vi "streams test.vi"() -> ()   [LabVIEW 2013, in "tag bus tests.lvlib"]
uses:
  tag bus tests.lvlib
  data stream/publisher/publish mode.ctl
  data stream/data stream definition.ctl
  data stream/data stream message type.ctl
  data stream/subscriber/enqueue mode.ctl
  data stream/subscriber/data bus stream subscriber.lvclass/data bus stream subscriber.ctl
  data stream/publisher/data bus stream publisher.lvclass
  data stream/subscriber/data bus stream subscriber.lvclass
panel:
  out "timed out? 3":bool
  out "timed out? 2":bool
  out "timed out?":bool
  out "Numeric 2":i32
  out "Numeric":i32
  out "error out":errorcluster
  in  "stream definition":T1
  out "element 2":T1
  out "element":T1
  in  "stop 3":bool
  in  "stop 2":bool
  in  "stop":bool
  in  "publish mode":T3
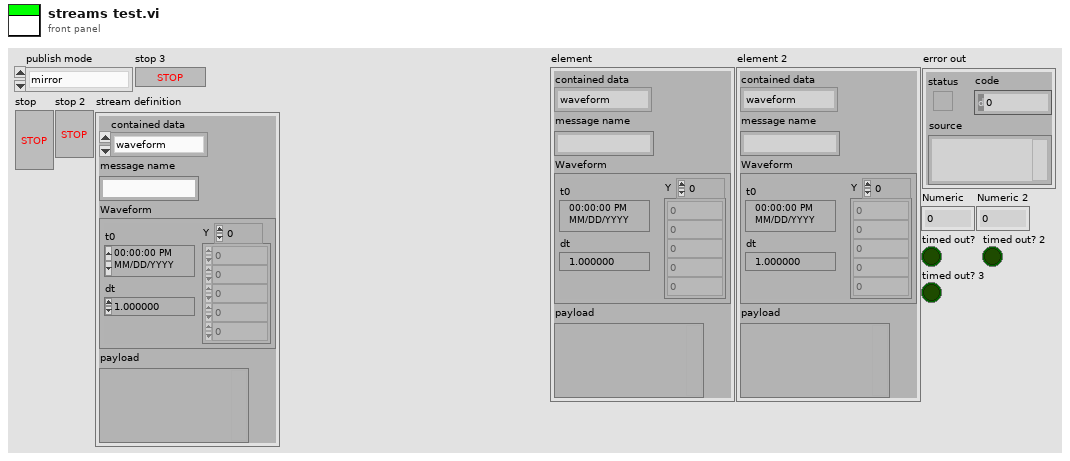
[diagram p1: front panel]
types:
  T1 = typedef "data stream definition.ctl" = cluster{"contained data":T2, "message name":string, "Waveform":waveform(dbl), "payload":variant}
  T2 = typedef "data stream message type.ctl" = enum16{"waveform", "message"}
  T3 = typedef "data bus stream publisher.lvclass/publish mode.ctl" = enum16{"mirror", "round robin"}
  T4 = typedef "data bus stream subscriber.lvclass/enqueue mode.ctl" = enum16{"lossy", "lossless"}
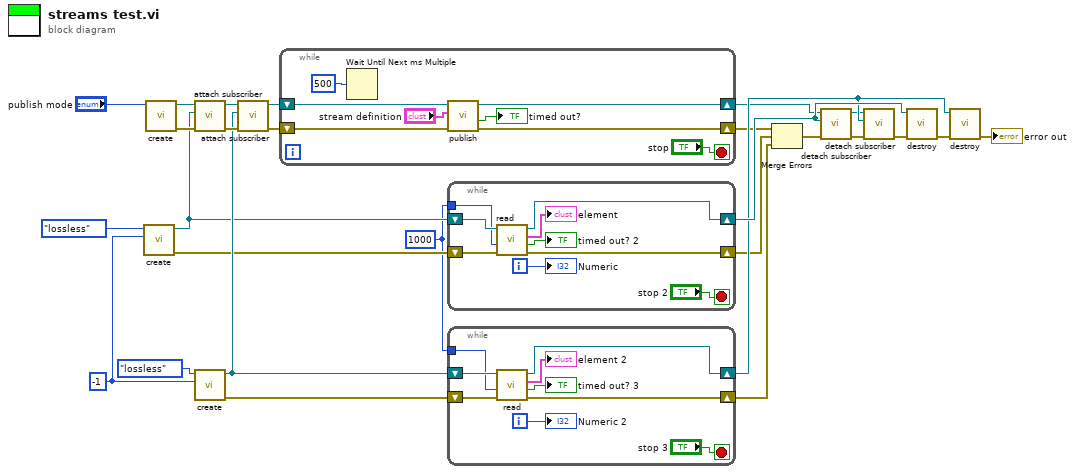
[diagram p0: block diagram]
diagram:
  w1 = 1000 ("timeout in ms (-1)")
  w2 = -1 ("max queue size (50)")
  n1 = call "create.vi"("max queue size (50)"=w2, "enqueue mode"=enqueue_mode."lossless") -> ("error out"=w4:errorcluster, "stream publisher out"=w19:refnum<class "data bus stream subscriber.lvclass">)  [unwired: 8 in]
  n2 = call "create.vi"("publish mode"="publish mode") -> ("error out"=w23:errorcluster, "stream publisher out"=w24:refnum<class "data bus stream publisher.lvclass">)  [unwired: 9 in]
  n3 = call "attach subscriber.vi"("error in"=w23, "stream publisher"=w19, "stream publisher in"=w24) -> ("error out"=w22:errorcluster, "stream publisher out"=w21:refnum<class "data bus stream publisher.lvclass">)  [unwired: 7 in]
  n4 = call "create.vi"("max queue size (50)"=w2, "enqueue mode"=enqueue_mode."lossless") -> ("error out"=w3:errorcluster, "stream publisher out"=w20:refnum<class "data bus stream subscriber.lvclass">)  [unwired: 8 in]
  n5 = call "attach subscriber.vi"("error in"=w22, "stream publisher"=w20, "stream publisher in"=w21) -> ("error out"=w10:errorcluster, "stream publisher out"=w13:refnum<class "data bus stream publisher.lvclass">)  [unwired: 7 in]
  n6 = while {
    shift-right: [w29] -> w9
    shift-left: w10 -> [w30]
    shift-right: [w32] -> w12
    shift-left: w13 -> [w33]
    stop <- "stop" stop-if-true
    n7 = Wait Until Next ms Multiple(millisecond multiple=u32 500) -> ()  [unwired: 1 out]
    n8 = call "publish.vi"("error in"=w30, "stream definition"="stream definition", "stream publisher in"=w33) -> ("error out"=w29:errorcluster, "timed out?"=→"timed out?":bool, "stream publisher out"=w32:refnum<class "data bus stream publisher.lvclass">)  [unwired: 6 in]
  }
  n9 = while {
    shift-right: [w40] -> w5
    shift-left: w4 -> [w39]
    shift-right: [w41] -> w18
    shift-left: w19 -> [w43]
    tunnel: w1 -> [w37]
    i -> [w38]
    stop <- "stop 2" stop-if-true
    n10 = call "read.vi"("error in"=w39, "timeout in ms (-1)"=w37, "stream publisher in"=w43) -> ("error out"=w40:errorcluster, "timed out?"=→"timed out? 2":bool, "element"=→"element":T1, "stream publisher out"=w41:refnum<class "data bus stream subscriber.lvclass">)  [unwired: 5 in]
    "Numeric" <- w38
  }
  n11 = while {
    shift-right: [w49] -> w6
    shift-left: w3 -> [w48]
    shift-right: [w50] -> w17
    shift-left: w20 -> [w52]
    tunnel: w1 -> [w46]
    i -> [w47]
    stop <- "stop 3" stop-if-true
    n12 = call "read.vi"("error in"=w48, "timeout in ms (-1)"=w46, "stream publisher in"=w52) -> ("error out"=w49:errorcluster, "timed out?"=→"timed out? 3":bool, "element"=→"element 2":T1, "stream publisher out"=w50:refnum<class "data bus stream subscriber.lvclass">)  [unwired: 5 in]
    "Numeric 2" <- w47
  }
  n13 = Merge Errors(w9, w5, w6) -> (w8:errorcluster)
  n14 = call "detach subscriber.vi"("error in"=w8, "stream publisher"=w18, "stream publisher in"=w12) -> ("error out"=w16:errorcluster, "stream publisher out"=w11:refnum<class "data bus stream publisher.lvclass">)  [unwired: 7 in]
  n15 = call "detach subscriber.vi"("error in"=w16, "stream publisher"=w17, "stream publisher in"=w11) -> ("error out"=w15:errorcluster)  [unwired: 7 in, 1 out]
  n16 = call "destroy.vi"("error in"=w15, "stream publisher in"=w18) -> ("error out"=w14:errorcluster)  [unwired: 9 in]
  n17 = call "destroy.vi"("error in"=w14, "stream publisher in"=w17) -> ("error out"=→"error out":errorcluster)  [unwired: 9 in]
